vi "SetSelectedPropertyAndValue.vi"(8 "error in (no error)":errorcluster, 9 "PropertyValue":variant, 10 "PropertyHierarchy":string[](array[string]), 11 "MetaDriver_v1 in":refnum<class "MetaDriver_v1.lvclass">) -> (0 "error out":errorcluster, 3 "MetaDriver_v1 out":refnum<class "MetaDriver_v1.lvclass">)   [LabVIEW 2020, in "MetaDriver_v1.lvclass"]
doc: "Set the currently selected property and specify it's new value"
uses:
  MetaDriver_v1.lvclass
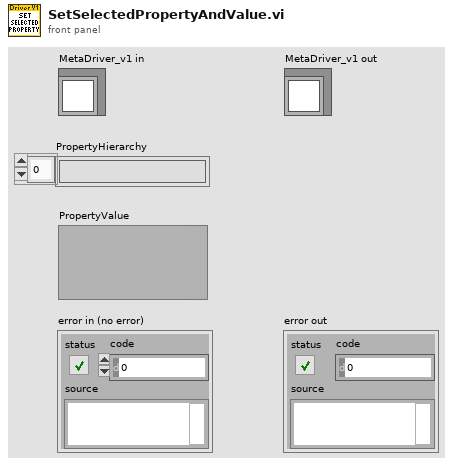
[diagram p1: front panel]
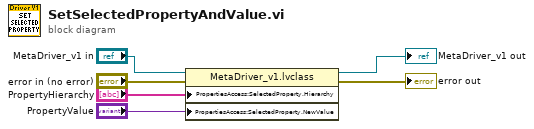
[diagram p0: block diagram]
diagram:
  n1 = property class="MetaDriver_v1.lvclass"(reference="MetaDriver_v1 in", error in="error in (no error)", "PropertiesAccess:SelectedProperty.Hierarchy"="PropertyHierarchy", "PropertiesAccess:SelectedProperty.NewValue"="PropertyValue") -> (reference out=→"MetaDriver_v1 out":refnum<class "MetaDriver_v1.lvclass">, error out=→"error out":errorcluster)
